vi "写入连接错误.vi"(8 "error in (no error)":errorcluster caption="错误输入（无错误）", 10 "连接错误":errorcluster, 11 "LS-H600-TCP Client输入":refnum<class "LS-H600-TCP Client.lvclass">) -> (0 "error out":errorcluster caption="错误输出", 3 "LS-H600-TCP Client输出":refnum<class "LS-H600-TCP Client.lvclass">)   [LabVIEW 2022 SP3, in "LS-H600-TCP Client.lvlib" / "LS-H600-TCP Client.lvclass"]
uses:
  LS-H600-TCP Client.lvclass
  LS-H600-TCP Client.lvclass/LS-H600-TCP Client.ctl
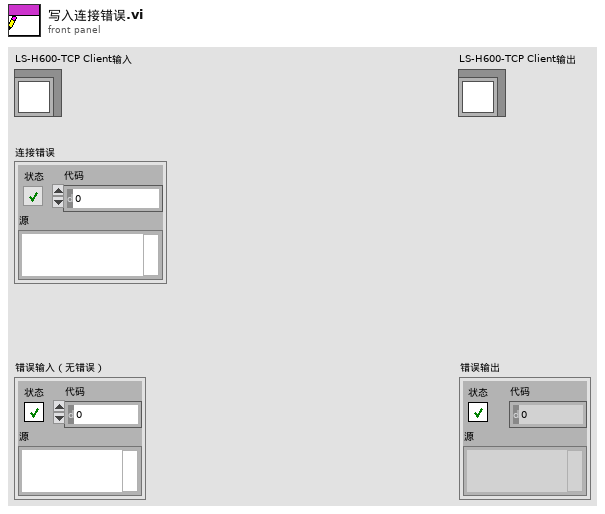
[diagram p1: front panel]
types:
  T1 = cluster{"数据输出":string, "data":cluster{"时间":timestamp, "仪器水深":dbl, "水温":dbl, "流速":dbl, "过水面积":dbl, "瞬时流量":dbl, "累积流量":dbl, "剖面流速":dbl[]}, "连接错误":errorcluster}
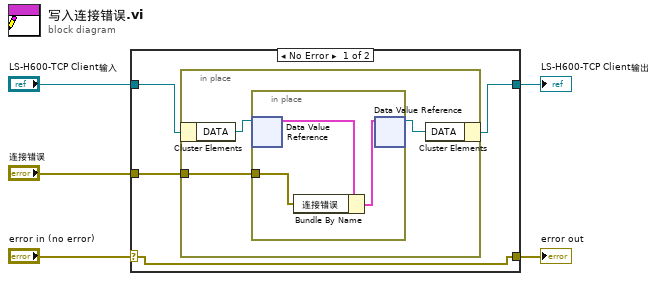
[diagram p0: block diagram]
diagram:
  n1 = case shown="No Error" "error in (no error)" {
    selector: "error in (no error)" -> [w7 w16]
    tunnel: [w7 w16] -> w4
    tunnel: [w8 w17] -> w2
    tunnel: "LS-H600-TCP Client输入" -> [w9 w17]
    tunnel: "连接错误" -> [w6 _]
    frame No Error {
      n2 = in-place {
        in-place-border: w6 -> [w10]
        n3 = in-place-cluster #1(w9) -> ("DATA"=w12:refnum<data-value>)
        n4 = in-place {
          in-place-border: w10 -> [w13]
          n5 = in-place-dvr #2(w12) -> (w15:T1)  [unwired: 1 out]
          n6 = Bundle By Name(cluster=w15, "连接错误"=w13) -> (w14:T1)
          n7 = in-place-dvr #2(w14) -> (w11:refnum<data-value>)  [unwired: 1 out]
        }
        n8 = in-place-cluster #1("DATA"=w11) -> (w8:refnum<class "LS-H600-TCP Client.lvclass">)
      }
    }
    frame Error {
    }
  }
  "error out" <- w4
  "LS-H600-TCP Client输出" <- w2
